vi "Initialise Directors.vi"(8 "error in (no error)":errorcluster, 10 "Internal Message Queue":refnum<queue>, 11 "InteractionProcessor in":refnum<class "InteractionProcessor.lvclass">) -> (0 "error out":errorcluster, 3 "InteractionProcessor out":refnum<class "InteractionProcessor.lvclass">)   [LabVIEW 2023, in "HAF.lvlib" / "InteractionProcessor.lvclass"]
doc: "Initialises all the Command Directors that have been given to the Test Processor."
uses:
  InteractionProcessor.lvclass
  Message.ctl
  All Internal Message Ids.ctl
  CommandDirector/CommandDirector.lvclass
  InteractionProcessor.lvclass/InteractionProcessor.ctl
  HAF.lvlib
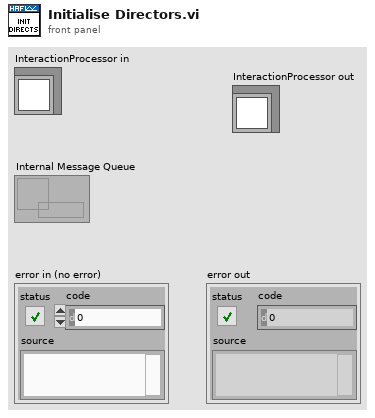
[diagram p1: front panel]
types:
  T1 = typedef "HAF.lvlib/All Internal Message Ids.ctl" = cluster{"Initialise":string, "Process":string, "Continue":string, "Done":string, "Pause":string, "Resume":string, "Stop":string, "Exit":string, "Inject":string}
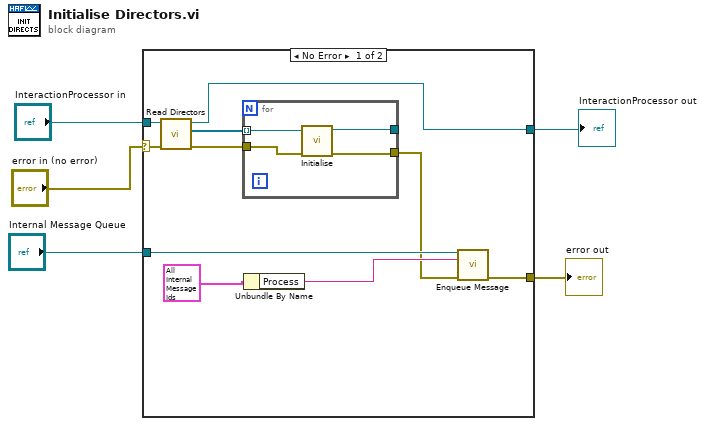
[diagram p0: block diagram]
diagram:
  n1 = case shown="No Error" "error in (no error)" {
    selector: "error in (no error)" -> [w8 w20]
    tunnel: "InteractionProcessor in" -> [w15 w21]
    tunnel: [w14 w20] -> w4
    tunnel: "Internal Message Queue" -> [w11 _]
    tunnel: [w6 w21] -> w1
    frame No Error {
      n2 = call-dynamic "Read Directors.vi"("error in (no error)"=w8, "InteractionProcessor in"=w15) -> ("error out"=w10:errorcluster, "Directors"=w9:refnum<class "CommandDirector.lvclass">[], "InteractionProcessor out"=w6:refnum<class "InteractionProcessor.lvclass">)  [unwired: 7 in]
      n3 = for {
        tunnel: w9 -> [w19] mode=indexing
        tunnel: w10 -> [w18]
        tunnel: [w17] -> w7
        tunnel: [w16] -> _
        n4 = call-dynamic "Initialise.vi"("error in (no error)"=w18, "CommandDirector in"=w19) -> ("error out"=w17:errorcluster, "CommandDirector out"=w16:refnum<class "CommandDirector.lvclass">)  [unwired: 8 in]
      }
      n5 = Unbundle By Name(T1 {"Initialise"="Initialise", "Process"="Process", "Continue"="Continue", "Done"="Done", "Pause"="Pause", "Resume"="Resume", "Stop"="Stop", "Exit"="Exit", "Inject"=""} ("Message Ids")) -> ("Process"=w13:string)
      n6 = call "Enqueue Message.vi"("Message Queue In"=w11, "Message Id"=w13, "error in (no error)"=w7) -> ("error out"=w14:errorcluster)  [unwired: 11 in, 1 out]
    }
    frame Error {
    }
  }
  "error out" <- w4
  "InteractionProcessor out" <- w1
